vi "Build Start Stop Relationship Graph.vi"(11 "Links Info":T1[](array[typedef])) -> (3 "Graph":string)   [LabVIEW 2021, in "TAF Proj Document Type.lvlib" / "Dqmh Module.lvclass"]
uses:
  <vilib>/Wovalab/AntiDoc/Document Type/Add-ons/LabVIEW TAF Project/Dqmh Module/Dqmh Module.lvclass
  <vilib>/Wovalab/AntiDoc/Document Type/Add-ons/LabVIEW TAF Project/Dqmh Module/Event Callers--cluster.ctl
  <vilib>/Wovalab/AntiDoc/GraphBuilder/Renderer/Graphviz/Graphviz.lvclass
  C:/Program Files (x86)/National Instruments/LabVIEW 2021/vi.lib/Wovalab/AntiDoc/GraphBuilder/Renderer/Renderer.lvclass
  <vilib>/Wovalab/AntiDoc/GraphBuilder/Graph/Graph.lvclass
  <vilib>/Wovalab/AntiDoc/GraphBuilder/Shapes/Edge/Graphviz/Graphviz Edge Shape.lvclass
  <vilib>/Wovalab/AntiDoc/GraphBuilder/Shapes/Node/Graphviz/Graphviz Node Shape.lvclass
  <vilib>/Wovalab/AntiDoc/GraphBuilder/Shapes/Edge/Graphviz/Shape.ctl
  <vilib>/Wovalab/AntiDoc/GraphBuilder/Shapes/Edge/Graphviz/Colors.ctl
  <vilib>/Wovalab/AntiDoc/GraphBuilder/Shapes/Node/Graphviz/Colors.ctl
  <vilib>/Wovalab/AntiDoc/GraphBuilder/Shapes/Node/Graphviz/Shape.ctl
  <vilib>/Wovalab/AntiDoc/GraphBuilder/Renderer/Graphviz/Specific Node Shape Def.ctl
  <vilib>/Wovalab/AntiDoc/GraphBuilder/Renderer/Graphviz/Specific Edge Shape Def.ctl
  <vilib>/Wovalab/AntiDoc/GraphBuilder/Renderer/Graphviz/Graph Direction.ctl
  <vilib>/Wovalab/AntiDoc/GraphBuilder/Edge/Edge.lvclass
  <vilib>/Wovalab/AntiDoc/GraphBuilder/Node/Node.lvclass
  <vilib>/Wovalab/AntiDoc/Document Type/Add-ons/LabVIEW TAF Project/TAF Proj Document Type.lvlib
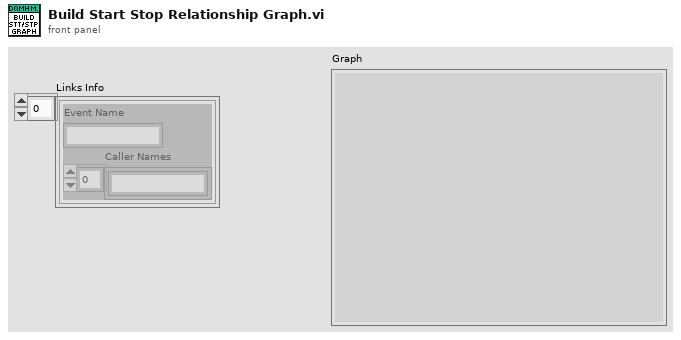
[diagram p1: front panel]
types:
  T1 = typedef "TAF Proj Document Type.lvlib/Dqmh Module.lvclass/Event Callers--cluster.ctl" = cluster{"Event Name":string, "Caller Names":string[]}
  T2 = typedef "GraphBuilder.lvlib/Graphviz.lvclass/Graph Direction.ctl" = enum16{"Top to Bottom", "Left To Right", "Bottom to Top", "Right to Left"}
  T3 = typedef "GraphBuilder.lvlib/Graphviz.lvclass/Specific Edge Shape Def.ctl" = cluster{"Source Node ID":string, "Target Node ID":string, "Caption":string, "Graphviz Edge Shape":refnum<class "Graphviz Edge Shape.lvclass">}
  T4 = typedef "GraphBuilder.lvlib/Graphviz.lvclass/Specific Node Shape Def.ctl" = cluster{"Node ID":string, "Graphviz Node Shape":refnum<class "Graphviz Node Shape.lvclass">}
  T5 = typedef "GraphBuilder.lvlib/Graphviz Node Shape.lvclass/Shape.ctl" = enum16{"box", "polygon", "ellipse", "oval", "circle", "point", "egg", "triangle", "plaintext", "plain", "diamond", "trapezium", "parallelogram", "house", "pentagon", "hexagon", "septagon", "octagon", "doublecircle", "doubleoctagon", "tripleoctagon", "invtriangle", "invtrapezium", "invhouse", "Mdiamond", "Msquare", "Mcircle", "rect", "rectangle", "square", "star", "none", "underline", "cylinder", "note", "tab", "folder", "box3D", "component", "promoter", "cds", "terminator", "utr", "primersite", "restrictionsite", "fivepoverhang", "threepoverhang", "noverhang", "assembly", "signature", "insulator", "ribosite", "rnastab", "proteasesite", "proteinstab", "rpromoter", "rarrow", "larrow", "lpromoter"}
  T6 = typedef "GraphBuilder.lvlib/Graphviz Node Shape.lvclass/Colors.ctl" = enum16{"aliceblue", "antiquewhite", "aqua", "aquamarine", "azure", "beige", "bisque", "black", "blanchedalmond", "blue", "blueviolet", "brown", "burlywood", "cadetblue", "chartreuse", "chocolate", "coral", "cornflowerblue", "cornsilk", "crimson", "cyan", "darkblue", "darkcyan", "darkgoldenrod", "darkgray", "darkgreen", "darkgrey", "darkkhaki", "darkmagenta", "darkolivegreen", "darkorange", "darkorchid", "darkred", "darksalmon", "darkseagreen", "darkslateblue", "darkslategray", "darkslategrey", "darkturquoise", "darkviolet", "deeppink", "deepskyblue", "dimgray", "dimgrey", "dodgerblue", "firebrick", "floralwhite", "forestgreen", "fuchsia", "gainsboro", "ghostwhite", "gold", "goldenrod", "gray", "green", "greenyellow", "grey", "honeydew", "hotpink", "indianred", "indigo", "ivory", "khaki", "lavender", "lavenderblush", "lawngreen", "lemonchiffon", "lightblue", "lightcoral", "lightcyan", "lightgoldenrodyellow", "lightgray", "lightgreen", "lightgrey", "lightpink", "lightsalmon", "lightseagreen", "lightskyblue", "lightslategray", "lightslategrey", "lightsteelblue", "lightyellow", "lime", "limegreen", "linen", "magenta", "maroon", "mediumaquamarine", "mediumblue", "mediumorchid", "mediumpurple", "mediumseagreen", "mediumslateblue", "mediumspringgreen", "mediumturquoise", "mediumvioletred", "midnightblue", "mintcream", "mistyrose", "moccasin", "navajowhite", "navy", "oldlace", "olive", "olivedrab", "orange", "orangered", "orchid", "palegoldenrod", "palegreen", "paleturquoise", "palevioletred", "papayawhip", "peachpuff", "peru", "pink", "plum", "powderblue", "purple", "red", "rosybrown", "royalblue", "saddlebrown", "salmon", "sandybrown", "seagreen", "seashell", "sienna", "silver", "skyblue", "slateblue", "slategray", "slategrey", "snow", "springgreen", "steelblue", "tan", "teal", "thistle", "tomato", "turquoise", "violet", "wheat", "white", "whitesmoke", "yellow", "yellowgreen"}
  T7 = typedef "GraphBuilder.lvlib/Graphviz Edge Shape.lvclass/Colors.ctl" = enum16{"aliceblue", "antiquewhite", "aqua", "aquamarine", "azure", "beige", "bisque", "black", "blanchedalmond", "blue", "blueviolet", "brown", "burlywood", "cadetblue", "chartreuse", "chocolate", "coral", "cornflowerblue", "cornsilk", "crimson", "cyan", "darkblue", "darkcyan", "darkgoldenrod", "darkgray", "darkgreen", "darkgrey", "darkkhaki", "darkmagenta", "darkolivegreen", "darkorange", "darkorchid", "darkred", "darksalmon", "darkseagreen", "darkslateblue", "darkslategray", "darkslategrey", "darkturquoise", "darkviolet", "deeppink", "deepskyblue", "dimgray", "dimgrey", "dodgerblue", "firebrick", "floralwhite", "forestgreen", "fuchsia", "gainsboro", "ghostwhite", "gold", "goldenrod", "gray", "green", "greenyellow", "grey", "honeydew", "hotpink", "indianred", "indigo", "ivory", "khaki", "lavender", "lavenderblush", "lawngreen", "lemonchiffon", "lightblue", "lightcoral", "lightcyan", "lightgoldenrodyellow", "lightgray", "lightgreen", "lightgrey", "lightpink", "lightsalmon", "lightseagreen", "lightskyblue", "lightslategray", "lightslategrey", "lightsteelblue", "lightyellow", "lime", "limegreen", "linen", "magenta", "maroon", "mediumaquamarine", "mediumblue", "mediumorchid", "mediumpurple", "mediumseagreen", "mediumslateblue", "mediumspringgreen", "mediumturquoise", "mediumvioletred", "midnightblue", "mintcream", "mistyrose", "moccasin", "navajowhite", "navy", "oldlace", "olive", "olivedrab", "orange", "orangered", "orchid", "palegoldenrod", "palegreen", "paleturquoise", "palevioletred", "papayawhip", "peachpuff", "peru", "pink", "plum", "powderblue", "purple", "red", "rosybrown", "royalblue", "saddlebrown", "salmon", "sandybrown", "seagreen", "seashell", "sienna", "silver", "skyblue", "slateblue", "slategray", "slategrey", "snow", "springgreen", "steelblue", "tan", "teal", "thistle", "tomato", "turquoise", "violet", "wheat", "white", "whitesmoke", "yellow", "yellowgreen"}
  T8 = typedef "GraphBuilder.lvlib/Graphviz Edge Shape.lvclass/Shape.ctl" = enum16{"box", "lbox", "rbox", "obox", "olbox", "orbox", "crow", "lcrow", "rcrow", "diamond", "ldiamond", "rdiamond", "odiamond", "oldiamond", "ordiamond", "dot", "odot", "inv", "linv", "rinv", "oinv", "olinv", "orinv", "none", "normal", "lnormal", "rnormal", "onormal", "olnormal", "ornormal", "tee", "ltee", "rtee", "vee", "lvee", "rvee", "curve", "lcurve", "rcurve", "icurve", "licurve", "ricurve"}
  T9 = typedef "GraphBuilder.lvlib/Graphviz Edge Shape.lvclass/Style.ctl" = enum8{"filled", "invisible", "diagonals", "rounded", "dashed", "dotted", "solid", "bold"}
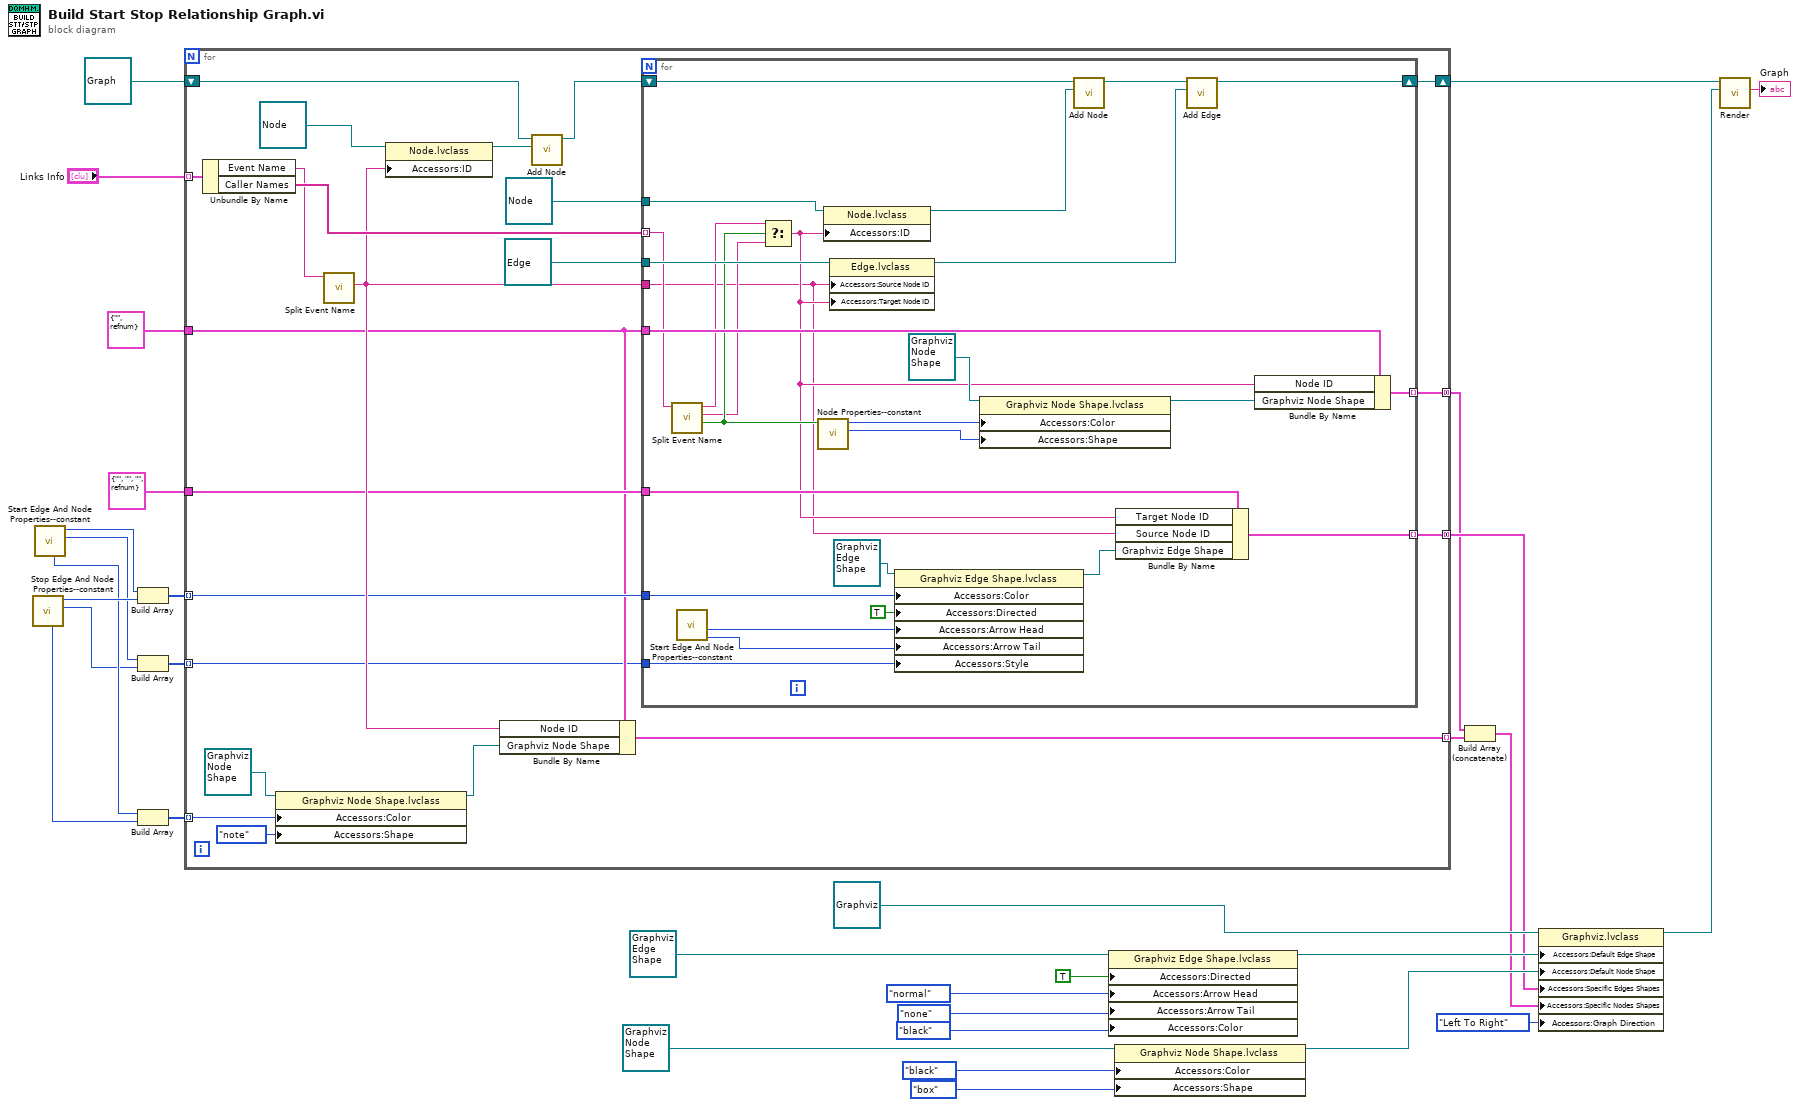
[diagram p0: block diagram]
diagram:
  n1 = call <vilib>:"Stop Edge And Node Properties--constant.vi"() -> ("Edge Style"=w2:T9, "Edge Color"=w8:T7, "Node Color"=w6:T6)  [unwired: 6 in, 3 out]
  n2 = call <vilib>:"Start Edge And Node Properties--constant.vi"() -> ("Edge Style"=w3:T9, "Edge Color"=w9:T7, "Node Color"=w5:T6)  [unwired: 6 in, 3 out]
  n3 = Build Array(w9, w8) -> (w7:T7[])
  n4 = Build Array(w3, w2) -> (w1:T9[])
  n5 = Build Array(w5, w6) -> (w4:T6[])
  n6 = for {
    tunnel: "Links Info" -> [w54] mode=indexing
    shift-right: [w49] -> w31
    shift-left: refnum<class "Graph.lvclass"> refnum ("GraphBuilder.lvlib:Graph.lvclass") -> [w53]
    tunnel: T4 {"Node ID"="", "Graphviz Node Shape"=refnum} ("Specific Node Shape") -> [w35]
    tunnel: [w41] -> w15 mode=indexing
    tunnel: w4 -> [w38] mode=indexing
    tunnel: T3 {"Source Node ID"="", "Target Node ID"="", "Caption"="", "Graphviz Edge Shape"=refnum} ("Specific Node Shape") -> [w39]
    tunnel: [w37] -> w13 mode=concatenating
    tunnel: w7 -> [w36] mode=indexing
    tunnel: [w34] -> w11 mode=concatenating
    tunnel: w1 -> [w33] mode=indexing
    n7 = Unbundle By Name(w54) -> ("Event Name"=w45:string, "Caller Names"=w51:string[])
    n8 = property class="Graphviz Node Shape.lvclass"(reference=refnum<class "Graphviz Node Shape.lvclass"> refnum ("GraphBuilder.lvlib:Graphviz Node Shape.lvclass"), "Accessors:Color"=w38, "Accessors:Shape"=Shape."note" ("Shape")) -> (reference out=w42:refnum<class "Graphviz Node Shape.lvclass">)  [unwired: 1 in, 1 out]
    n9 = call <vilib>:"Split Event Name.vi"("Event Name"=w45) -> ("Vi Name"=w44:string)  [unwired: 8 in, 2 out]
    n10 = property class="Node.lvclass"(reference=refnum<class "Node.lvclass"> refnum ("GraphBuilder.lvlib:Node.lvclass"), "Accessors:ID"=w44) -> (reference out=w52:refnum<class "Node.lvclass">)  [unwired: 1 in, 1 out]
    n11 = Bundle By Name(cluster=w35, "Node ID"=w44, "Graphviz Node Shape"=w42) -> (w41:T4)
    n12 = call-dynamic "Add Node.vi"("Node"=w52, "Graph in"=w53) -> ("Graph out"=w50:refnum<class "Graph.lvclass">)  [unwired: 8 in, 1 out]
    n13 = for {
      tunnel: w51 -> [w60] mode=indexing
      shift-right: [w77] -> w49
      shift-left: w50 -> [w82]
      tunnel: refnum<class "Node.lvclass"> refnum ("GraphBuilder.lvlib:Node.lvclass") -> [w81]
      tunnel: refnum<class "Edge.lvclass"> refnum ("GraphBuilder.lvlib:Edge.lvclass") -> [w79]
      tunnel: w44 -> [w55]
      tunnel: w39 -> [w75]
      tunnel: [w72] -> w37 mode=indexing
      tunnel: w36 -> [w70]
      tunnel: w35 -> [w68]
      tunnel: [w66] -> w34 mode=indexing
      tunnel: w33 -> [w59]
      n14 = call <vilib>:"Split Event Name.vi"("Event Name"=w60) -> ("Lvlib?"=w63:bool, "Vi Name"=w61:string, "Library Name"=w62:string)  [unwired: 8 in]
      n15 = call <vilib>:"Start Edge And Node Properties--constant.vi"() -> ("Edge Arrow Tail"=w57:T8, "Edge Arrow Head"=w58:T8)  [unwired: 6 in, 4 out]
      n16 = Select(t=w62, s=w63, f=w61) -> (s? t:f=w56:string)
      n17 = call <vilib>:"Node Properties--constant.vi"("Lvlib"=w63) -> ("Shape"=w64:T5, "Color"=w65:T6)  [unwired: 9 in]
      n18 = property class="Node.lvclass"(reference=w81, "Accessors:ID"=w56) -> (reference out=w80:refnum<class "Node.lvclass">)  [unwired: 1 in, 1 out]
      n19 = property class="Edge.lvclass"(reference=w79, "Accessors:Source Node ID"=w55, "Accessors:Target Node ID"=w56) -> (reference out=w76:refnum<class "Edge.lvclass">)  [unwired: 1 in, 1 out]
      n20 = property class="Graphviz Edge Shape.lvclass"(reference=refnum<class "Graphviz Edge Shape.lvclass"> refnum ("Graphviz Edge Shape"), "Accessors:Color"=w70, "Accessors:Directed"=TRUE ("Directed"), "Accessors:Arrow Head"=w58, "Accessors:Arrow Tail"=w57, "Accessors:Style"=w59) -> (reference out=w73:refnum<class "Graphviz Edge Shape.lvclass">)  [unwired: 1 in, 1 out]
      n21 = property class="Graphviz Node Shape.lvclass"(reference=refnum<class "Graphviz Node Shape.lvclass"> refnum ("GraphBuilder.lvlib:Graphviz Node Shape.lvclass"), "Accessors:Color"=w65, "Accessors:Shape"=w64) -> (reference out=w67:refnum<class "Graphviz Node Shape.lvclass">)  [unwired: 1 in, 1 out]
      n22 = call-dynamic "Add Node.vi"("Node"=w80, "Graph in"=w82) -> ("Graph out"=w78:refnum<class "Graph.lvclass">)  [unwired: 8 in, 1 out]
      n23 = Bundle By Name(cluster=w75, "Target Node ID"=w56, "Source Node ID"=w55, "Graphviz Edge Shape"=w73) -> (w72:T3)
      n24 = call-dynamic "Add Edge.vi"("Edge"=w76, "Graph in"=w78) -> ("Graph out"=w77:refnum<class "Graph.lvclass">)  [unwired: 8 in, 1 out]
      n25 = Bundle By Name(cluster=w68, "Node ID"=w56, "Graphviz Node Shape"=w67) -> (w66:T4)
    }
  }
  n26 = property class="Graphviz Edge Shape.lvclass"(reference=refnum<class "Graphviz Edge Shape.lvclass"> refnum ("GraphBuilder.lvlib:Graphviz Edge Shape.lvclass"), "Accessors:Directed"=TRUE ("Directed"), "Accessors:Arrow Head"=Shape."normal" ("Arrow Head"), "Accessors:Arrow Tail"=Shape."none" ("Arrow Tail"), "Accessors:Color"=Colors."black" ("Color")) -> (reference out=w27:refnum<class "Graphviz Edge Shape.lvclass">)  [unwired: 1 in, 1 out]
  n27 = property class="Graphviz Node Shape.lvclass"(reference=refnum<class "Graphviz Node Shape.lvclass"> refnum ("GraphBuilder.lvlib:Graphviz Node Shape.lvclass"), "Accessors:Color"=Colors."black" ("Color"), "Accessors:Shape"=Shape."box" ("Shape")) -> (reference out=w28:refnum<class "Graphviz Node Shape.lvclass">)  [unwired: 1 in, 1 out]
  n28 = Build Array (concatenate)(w11, w15) -> (w12:T4[])
  n29 = property class="Graphviz.lvclass"(reference=refnum<class "Graphviz.lvclass"> refnum ("GraphBuilder.lvlib:Graphviz.lvclass"), "Accessors:Default Edge Shape"=w27, "Accessors:Default Node Shape"=w28, "Accessors:Specific Edges Shapes"=w13, "Accessors:Specific Nodes Shapes"=w12, "Accessors:Graph Direction"=Graph_Direction."Left To Right" ("Graph Direction")) -> (reference out=w29:refnum<class "Graphviz.lvclass">)  [unwired: 1 in, 1 out]
  n30 = call-dynamic "Render.vi"("Renderer"=w29, "Graph in"=w31) -> ("Rendered Stream"=→"Graph":string)  [unwired: 7 in, 2 out]
